vi "ConnectionTest.vi"(3 "Tar letter":string="G", 4 "RunRobot":bool, 5 "Tug letter":string="P") -> (0 "Tug X":i32, 1 "Tug H":i32, 2 "Tug Y":i32)   [LabVIEW 2012]
panel:
  out "RECORDED TAR INFO":T1(array[cluster])
  out "RECORDED TUG INFO":T1(array[cluster])
  out "BS Time Out?":bool
  out "Valid ?":bool
  out "udp rate":bool
  out "RBI Size":dbl
  in  "WhereAmI?FromBase":T2
  out "Buoy locations":cluster{"regular expression":string, i32, i32}[](array[cluster])
  out "Base Station data rec'd":string
  in  "error in":errorcluster
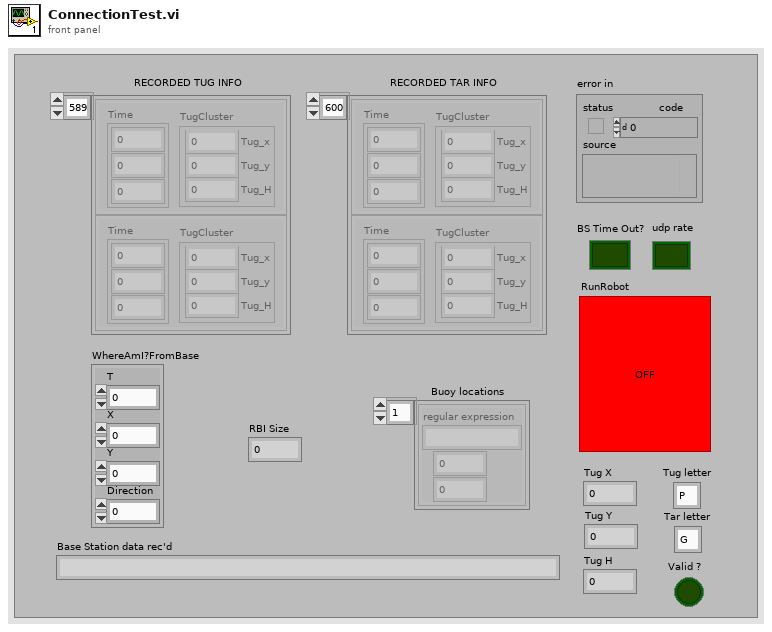
[diagram p1: front panel]
types:
  T1 = cluster{"TugCluster":cluster{"Tug_x":dbl, "Tug_y":dbl, "Tug_H":dbl}, "Time":cluster{i32, i32, i32}}[]
  T2 = cluster{"T":dbl, "X":dbl, "Y":dbl, "Direction":dbl}
  T3 = cluster{"regular expression":string, i32, i32, i32}
  T4 = cluster{"TarCluster":cluster{"Tar_x":dbl, "Tar_y":dbl, "Tar_H":dbl}, "Time":cluster{i32, i32, i32}}
  T5 = cluster{"TugCluster":cluster{"Tug_x":dbl, "Tug_y":dbl, "Tug_H":dbl}, "Time":cluster{i32, i32, i32}}
  T6 = cluster{"TarCluster":cluster{"Tar_x":dbl, "Tar_y":dbl, "Tar_H":dbl}, "Time":cluster{i32, i32, i32}}[]
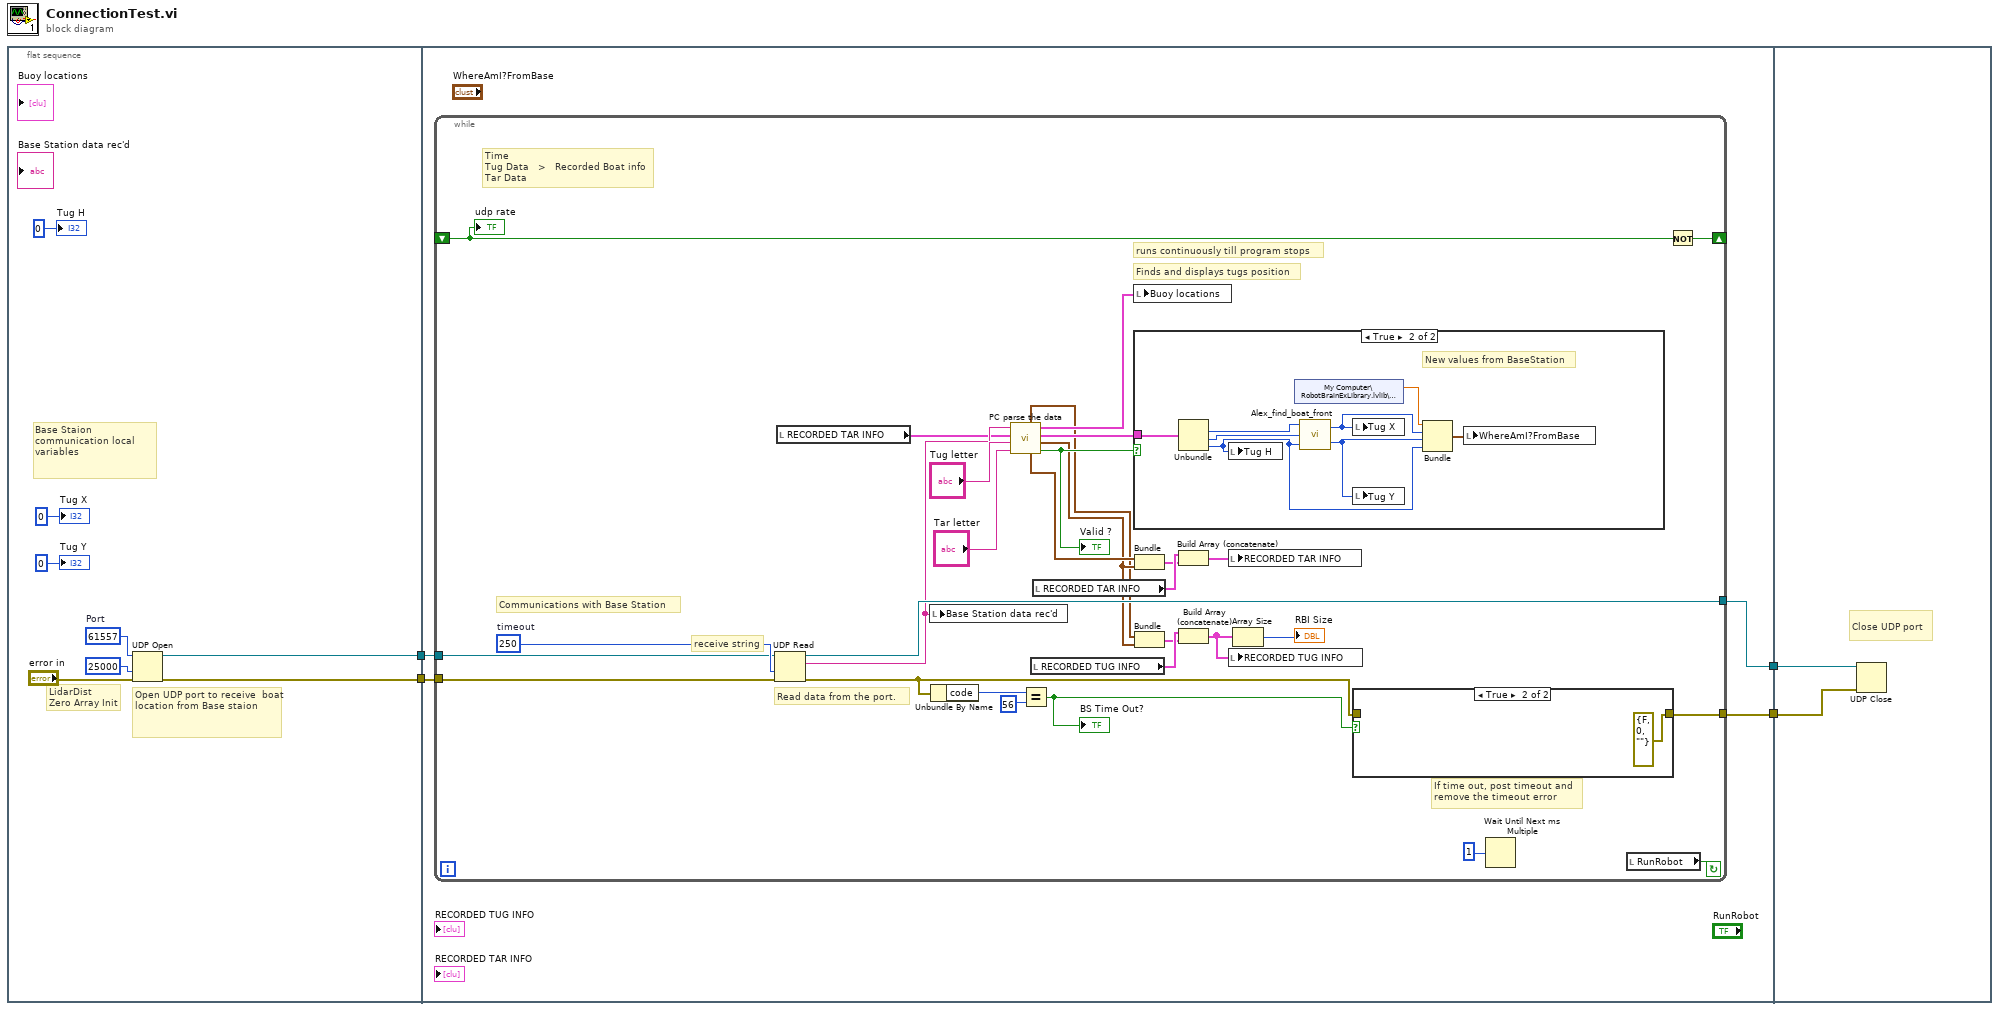
[diagram p0: block diagram]
diagram:
  n1 = flat-sequence {
    tunnel: [w6] -> w4
    tunnel: [w5] -> w3
    tunnel: w4 -> [w16]
    tunnel: w3 -> [w15]
    tunnel: [w14] -> w2
    tunnel: [w13] -> w1
    tunnel: w2 -> [w58]
    tunnel: w1 -> [w57]
    frame #0 {
      w12 = u16 61557  # Port
      # "LidarDist\nZero Array Init"
      # "Base Staion communication local variables"
      # "Open UDP port to receive  boat location from Base staion"
      n2 = UDP Open(8:"error in", 9:25000 ("timeout ms (25000)"), 11:w12) -> (port=w5:refnum<k16>, 0:w6:errorcluster)  [unwired: 2 in, 1 out]
      "Tug X" <- 0 ("Tug X")
      "Tug Y" <- 0 ("Tug Y")
      "Tug H" <- 0 ("Tug H")
    }
    frame #1 {
      n3 = while {
        tunnel: [w39] -> w13
        tunnel: [w38] -> w14
        shift-right: [w32] -> _
        shift-left: _ -> [w31]
        tunnel: w16 -> [w18]
        tunnel: w15 -> [w17]
        stop <- w40 continue-if-true
        w42 = 250  # timeout
        # "Time               \nTug Data   >   Recorded Boat info\nTar Data"
        # "Finds and displays tugs position"
        # "runs continuously till program stops"
        # "Communications with Base Station"
        # "receive string"
        # "If time out, post timeout and\nremove the timeout error"
        # "Read data from the port."
        n4 = UDP Read(connection ID=w17, timeout ms (25000)=w42, 8:w18) -> (data out=w33:string, error out=w43:errorcluster, 3:w38:refnum<k16>)  [unwired: 1 in, 2 out]
        n5 = local read "RECORDED TAR INFO"() -> (w19:T1)
        n6 = local write "Base Station data rec'd"(w33) -> ()
        n7 = Unbundle By Name(w43) -> ("code"=w46:i32)
        n8 = call "PC parse the data.vi"("Nav String"=w33, "RECORDED TAR INFO"=w19, "Tug"="Tug letter", "Tar"="Tar letter") -> ("TugCluster"=w22:cluster{"Tug_x":dbl, "Tug_y":dbl, "Tug_H":dbl}, "TarCluster"=w24:cluster{"Tar_x":dbl, "Tar_y":dbl, "Tar_H":dbl}, "Buoy locations"=w37:cluster{"regular expression":string, i32, i32}[], "Tug Location"=w35:T3, "Time"=w23:cluster{i32, i32, i32}, "Valid?"=w36:bool)
        "Valid ?" <- w36
        n9 = Equal?(x=w46, y=56) -> (x = y?=w44:bool)
        "BS Time Out?" <- w44
        n10 = local read "RECORDED TUG INFO"() -> (w29:T1)
        n11 = local read "RECORDED TAR INFO"() -> (w26:T1)
        n12 = local write "Buoy locations"(w37) -> ()
        n13 = case shown="True" w36 {
          tunnel: w35 -> [_ w54]
          frame False {
            # "No \nchange"
          }
          frame True {
            # "New values from BaseStation"
            n14 = Unbundle(w54) -> (w47:i32, w48:i32, w49:i32)  [unwired: 1 out]
            n15 = local write "Tug H"(w49) -> ()
            n16 = shared-variable "My Computer\\RobotBrainExLibrary.lvlib\\MissionTime"() -> (w53:dbl)  [unwired: 1 in, 1 out]
            n17 = call "Alex_find_boat_front.vi"("Heading"=w49, "Y"=w48, "X"=w47) -> ("Y"=w51:i32, "X"=w50:i32)
            n18 = local write "Tug X"(w50) -> ()
            n19 = local write "Tug Y"(w51) -> ()
            n20 = Bundle(w53, "X"=w50, "Y"=w51, w49) -> (w52:cluster{dbl, "X":i32, "Y":i32, i32})  [unwired: 1 in]
            n21 = local write "WhereAmI?FromBase"(w52) -> ()
          }
        }
        n22 = Bundle("TarCluster"=w24, "Time"=w23) -> (w20:T4)  [unwired: 1 in]
        n23 = Bundle("TugCluster"=w22, "Time"=w23) -> (w21:T5)  [unwired: 1 in]
        n24 = Build Array (concatenate)(w26, w20) -> (w25:T6)
        n25 = Build Array (concatenate)(w29, w21) -> (w28:T1)
        n26 = local write "RECORDED TAR INFO"(w25) -> ()
        n27 = local write "RECORDED TUG INFO"(w28) -> ()
        n28 = Array Size(array=w28) -> (size(s)=→"RBI Size":i32)
        n29 = case shown="True" w44 {
          tunnel: [w55 errorcluster {"status"=FALSE, "code"=0, "source"=""} ("error out")] -> w39
          tunnel: w43 -> [w55 _]
          frame False {
          }
          frame True {
          }
        }
        n30 = Wait Until Next ms Multiple(millisecond multiple=u32 1) -> ()  [unwired: 1 out]
        n31 = local read "RunRobot"() -> (w40:bool)
        n32 = Not(x=w31) -> (.not. x?=w32:bool)
        "udp rate" <- w31
      }
    }
    frame #2 {
      # "Close UDP port"
      n33 = UDP Close(connection ID=w58, 8:w57) -> ()  [unwired: 2 out]
    }
  }
